vi "SET_mech.vi"() -> ()   [LabVIEW 2013]
uses:
  <instrlib>/niScope/Controls/niScope trigger slope.ctl
  <instrlib>/niScope/Controls/niScope trigger coupling.ctl
  <instrlib>/niScope/Configure/Trigger/niScope Configure Trigger Edge.vi
  <vilib>/Waveform/WDTFileIO.llb/Export Waveforms To Spreadsheet File (1D).vi
panel:
  in  "stop":bool
  out "instrument handle out":refnum<k15>="PXI1Slot2"
  in  "negative(T)/positive pulse(F)":bool
  out "the value of the waveform":dbl=1.6544701748989392 format="%0.2f"
  out "Waveform Graph":waveform(dbl)[](graph)=[{"t0"=timestamp(3536397918.132065 s since 1904-01-01), "dt"=2e-08, "Y"=array[10000 elements]}]
  in  "timeout (s)":dbl caption="Timeout(s)" format="%.2f"
  in  "vertical range value":dbl=3.0 caption="Vertical Range (V)" format="%.2f"
  out "Папкец":path=path "C:/Users/user/Desktop/OSC/SET_mech/23  14_45_05"
  in  "Писать осциллограммы(T)/Нет(F)":bool
  in  "Path_for_write":path=path "C:/Users/user/Desktop/OSC/SET_mech"
  in  "min sample rate":dbl=50000000.0 format="%#_13p"
  in  "resource name":refnum<k15>="PXI1Slot2" caption="Resource Name"
  in  "channel name":string="0" caption="Channel Name(s)"
  in  "probe attenuation":dbl=10.0 caption="Probe Attenuation" format="%.1f"
  in  "trigger source":string(combo)="0" caption="Trigger Source"
  in  "reference position":dbl=10.0 caption="Ref Position" format="%.1f"
  in  "trigger level":dbl=1.0 caption="Trigger Level" format="%.2f"
  in  "trigger slope":T1 caption="Trigger Slope"
  in  "min record length":i32=10000 caption="Min. Record Length"
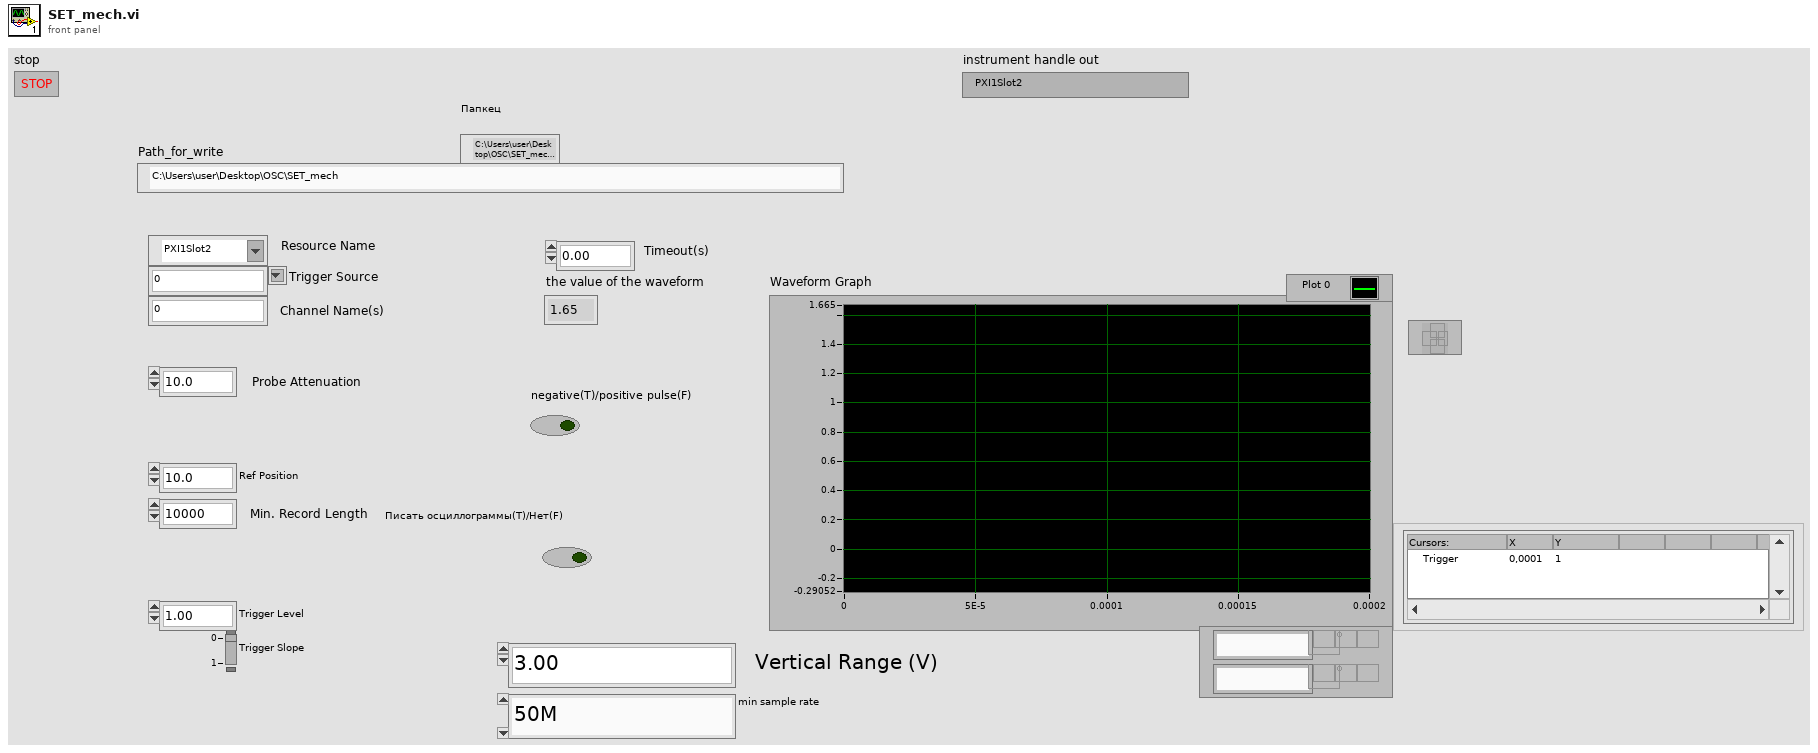
[diagram p1: front panel]
types:
  T1 = typedef "niScope trigger slope.ctl" = i32
  T2 = typedef "niScope trigger coupling.ctl" = u16
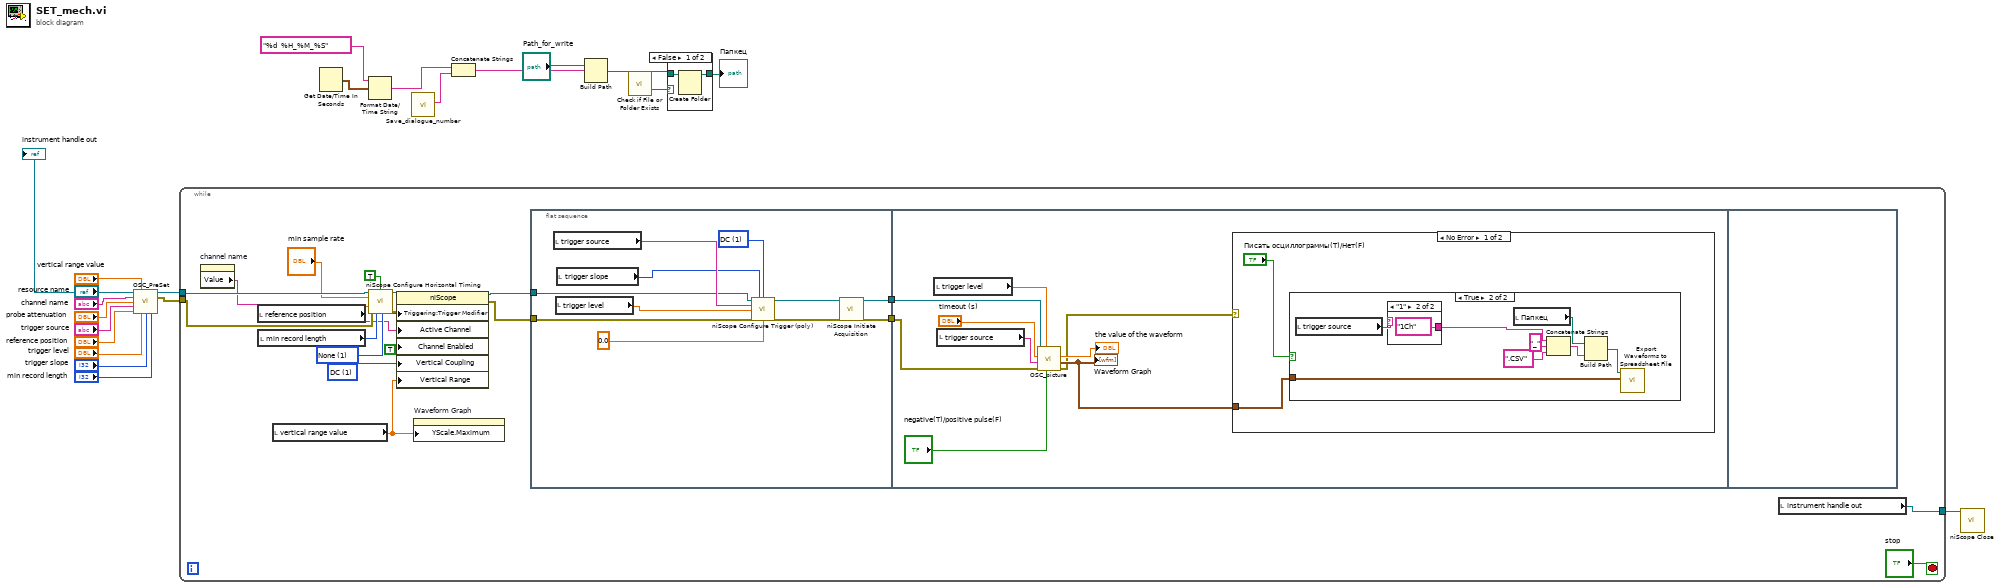
[diagram p0: block diagram]
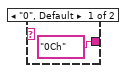
[diagram p3: hidden frame]
diagram:
  n1 = call "OSC_PreSet.vi"("resource name"="resource name", "vertical range"="vertical range value", "channel name"="channel name", "probe attenuation"="probe attenuation", "trigger source"="trigger source", "reference position"="reference position", "trigger level"="trigger level", "trigger slope"="trigger slope", "min record length"="min record length") -> ("instrument handle out"=w3:refnum<k15>, "error out"=w5:errorcluster)  [unwired: 5 in]
  "instrument handle out" <- w3
  n2 = while {
    tunnel: w5 -> [w39]
    tunnel: w3 -> [w38]
    tunnel: [w23] -> w1
    stop <- "stop" stop-if-true
    w28 = 1 items=["AC", "DC", "Ground"] ("Vertical:Vertical Coupling")
    w35 = 1 items=["None"=1, "Auto Trigger"=2] ("trigger modifier")
    n3 = property on="channel name" class="Str"() -> ("Value"=w29:string)  [unwired: 2 in, 2 out]
    n4 = local read "reference position"() -> (w36:dbl)
    n5 = local read "min record length"() -> (w37:i32)
    n6 = local read "vertical range value"() -> (w25:dbl)
    n7 = call <instrlib>:"niScope Configure Horizontal Timing.vi"("instrument handle"=w38, "enforce realtime"=TRUE, "min sample rate"="min sample rate", "reference position"=w36, "error in"=w39, "min record length"=w37) -> ("instrument handle out"=w32:refnum<k15>, "error out"=w33:errorcluster)  [unwired: 8 in]
    n8 = property class="niScope"(reference=w32, error in=w33, "Triggering:Trigger Modifier"=w35, "Active Channel"=w29, "Channel Enabled"=TRUE ("Vertical:Channel Enabled"), "Vertical Coupling"=w28, "Vertical Range"=w25) -> (reference out=w27:refnum<k15>, error out=w26:errorcluster)
    n9 = property on="Waveform Graph" class="WFGraph (strict)"("YScale.Maximum"=w25) -> ()  [unwired: 2 in, 2 out]
    n10 = flat-sequence {
      tunnel: w27 -> [w45]
      tunnel: w26 -> [w44]
      tunnel: [w43] -> w41
      tunnel: [w42] -> w40
      tunnel: w41 -> [w57]
      tunnel: w40 -> [w56]
      frame #0 {
        w49 = T2 1 items=["AC"=0, "DC"=1, "HF Reject"=3, "LF Reject"=4, "AC Plus HF Reject"=1001] ("trigger coupling")
        n11 = local read "trigger source"() -> (w52:string)
        n12 = local read "trigger level"() -> (w48:dbl)
        n13 = local read "trigger slope"() -> (w51:T1)
        n14 = call-poly <instrlib>:"niScope Configure Trigger (poly).vi"("instrument handle"=w45, "trigger slope"=w51, "trigger coupling"=w49, "trigger source"=w52, "trigger level"=w48, "error in"=w44, "trigger delay"=0.0) -> ("instrument handle out"=w47:refnum<k15>, "error out"=w46:errorcluster)  [unwired: 7 in]
        n15 = call <instrlib>:"niScope Initiate Acquisition.vi"("instrument handle"=w47, "error in"=w46) -> ("instrument handle out"=w43:refnum<k15>, "error out"=w42:errorcluster)  [unwired: 12 in]
      }
      frame #1 {
        n16 = local read "trigger level"() -> (w54:dbl)
        n17 = local read "trigger source"() -> (w59:string)
        n18 = call "OSC_picture.vi"("Falling(T)/Rising(F)"="negative(T)/positive pulse(F)", "trig level"=w54, "error in (no error)"=w56, "channels"=w59, "timeout (s) 2"="timeout (s)", "instrument handle"=w57) -> ("error out"=w55:errorcluster, "Waveform Graph"=w61:waveform(dbl)[], "the value of the waveform"=→"the value of the waveform":dbl)  [unwired: 2 in, 1 out]
        "Waveform Graph" <- w61
        n19 = case shown="No Error" w55 {
          tunnel: w61 -> [w62 _]
          frame No Error {
            n20 = case shown="True" "Писать осциллограммы(T)/Нет(F)" {
              tunnel: w62 -> [_ w69]
              frame False {
              }
              frame True {
                n21 = local read "trigger source"() -> (w66:string)
                n22 = case shown="\"1\"" w66 {
                  tunnel: ["0Ch" ("string") "1Ch" ("string")] -> w65
                  frame "0", Default {
                  }
                  frame "1" {
                  }
                }
                n23 = local read "Папкец"() -> (w68:path)
                n24 = Concatenate Strings(w65, "_" ("string"), ".CSV" ("string")) -> (w71:string)
                n25 = Build Path(base path=w68, name or relative path=w71) -> (appended path=w70:path)
                n26 = call-poly <vilib>:"Export Waveforms to Spreadsheet File.vi"("waveforms"=w69, "file path (dialog if empty)"=w70) -> ()  [unwired: 8 in, 2 out]
              }
            }
          }
          frame Error {
          }
        }
      }
      frame #2 {
      }
    }
    n27 = local read "instrument handle out"() -> (w23:refnum<k15>)
  }
  n28 = Get Date/Time In Seconds() -> (seconds since 1Jan1904=w17:timestamp)
  n29 = Format Date/Time String(time format string (%c)="%d  %H_%M_%S", seconds (now)=w17) -> (date/time string=w15:string)  [unwired: 1 in]
  n30 = call "Save_dialogue_number.vi"() -> ("Что делаем? Номер образца? 2"=w14:string)  [unwired: 10 in]
  n31 = Concatenate Strings(w15, w14) -> (w13:string)
  n32 = Build Path(base path="Path_for_write", name or relative path=w13) -> (appended path=w22:path)
  n33 = call <vilib>:"Check if File or Folder Exists.vi"("path"=w22) -> ("file or folder exists?"=w20:bool, "dup path"=w21:path)  [unwired: 8 in, 1 out]
  n34 = case shown="False" w20 {
    tunnel: w21 -> [w75 w76]
    tunnel: [w74 w76] -> w18
    frame False {
      n35 = Create Folder(path (use dialog)=w75) -> (created path=w74:path)  [unwired: 2 in, 2 out]
    }
    frame True {
    }
  }
  "Папкец" <- w18
  n36 = call <instrlib>:"niScope Close.vi"("instrument handle"=w1) -> ()  [unwired: 14 in, 1 out]
